vi "Register ROI group clicked on.vi"(6 "Value signalling? (F)":bool, 8 "error in (no error)":errorcluster, 10 "Valid":bool, 11 "Group index":i16) -> (0 "error out":errorcluster, 3 "Group index":i16)   [LabVIEW 2017]
uses:
  Global variables/gl_Functional Imaging-Global variables.vi
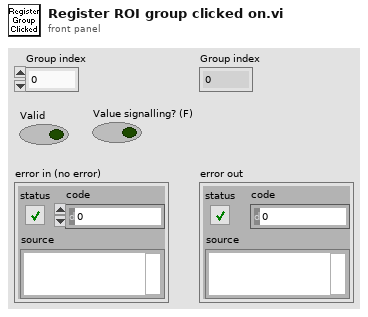
[diagram p1: front panel]
types:
  T1 = typedef "Functional Imging UI Refs.ctl" = cluster{"Menu ref":refnum<k9>, "Image control":refnum<vi>, "VI ref":refnum<vi>, "XGrapher":refnum<vi>, "Smoothing":refnum<vi>, "POI Averaging":refnum<vi>, "Normalize":refnum<vi>, "POI data points in each trial":refnum<vi>, "Channel":refnum<vi>, "Experiment data folder path":refnum<vi>, "[ROI vis]":refnum<vi>, "[Groups] visbl":T2, "Group Name":refnum<vi>, "POI index":refnum<vi>, "Trial No.":refnum<vi>, "Intensity Zoom":refnum<vi>, "Trial Cursor Enabled":refnum<vi>, "Number of Trials (ind 1)":refnum<vi>, "Number of Trials (ind 2)":refnum<vi>, "MiniScans Available":refnum<vi>, "POI Available":refnum<vi>, "Defer graph updates":refnum<vi>, "Waveform selector":refnum<vi>, "#of selected POI":refnum<vi>, "#of selected MiniScans":refnum<vi>, "#of selected groups":refnum<vi>, "Max Z-Projection":refnum<vi>, "Z-Plane Selector":refnum<vi>, "Index of miniscan point to visualise":refnum<vi>, "ROI vis. mode":refnum<vi>, "Total # of points":refnum<vi>, "Index of group clicked on":refnum<vi>, "Pane 1":refnum<vi>, "Pane 2":refnum<vi>, "Pane 3":refnum<vi>, "Pane 4":refnum<vi>, "Pane 5":refnum<vi>, "Pane 6":refnum<vi>, "Deselect all ROI":refnum<vi>, "Deselect all groups":refnum<vi>}
  T2 = typedef "Groups array referecne.ctl" = refnum<vi>
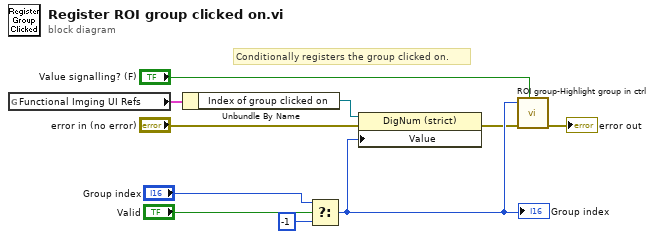
[diagram p0: block diagram]
diagram:
  # "Conditionally registers the group clicked on."
  n1 = global read "gl_Functional Imaging-Global variables.vi" "Functional Imging UI Refs"() -> (w10:T1)
  n2 = Unbundle By Name(w10) -> ("Index of group clicked on"=w9:refnum<vi>)
  n3 = Select(t="Group index", s="Valid", f=i16 -1) -> (s? t:f=w8:i16)
  "Group index" <- w8
  n4 = property on="Property Node" class="DigNum (strict)"(reference=w9, error in="error in (no error)", "Value"=w8) -> (error out=w3:errorcluster)  [unwired: 1 out]
  n5 = call "ROI group-Highlight group in ctrl.vi"("Value signalling?"="Value signalling? (F)", "error in (no error)"=w3, "Index of group to update"=w8) -> ("error out"=→"error out":errorcluster)  [unwired: 8 in]
